vi "Initialize.vi"(8 "error in (no error)":errorcluster caption="错误输入（无错误）", 11 "Generic输入":refnum<class "Generic.lvclass">) -> (0 "error out":errorcluster caption="错误输出", 3 "Generic输出":refnum<class "Generic.lvclass">)   [LabVIEW 2013, in "Hierarchy Framework.lvlib" / "Generic.lvclass"]
uses:
  Generic.lvclass
  Generic.lvclass/Generic.ctl
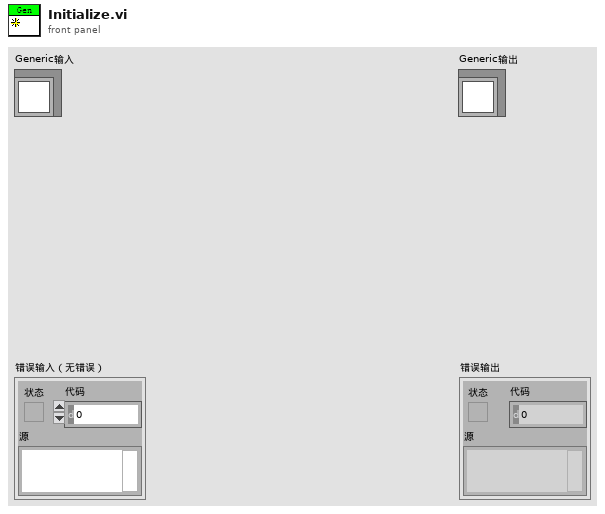
[diagram p1: front panel]
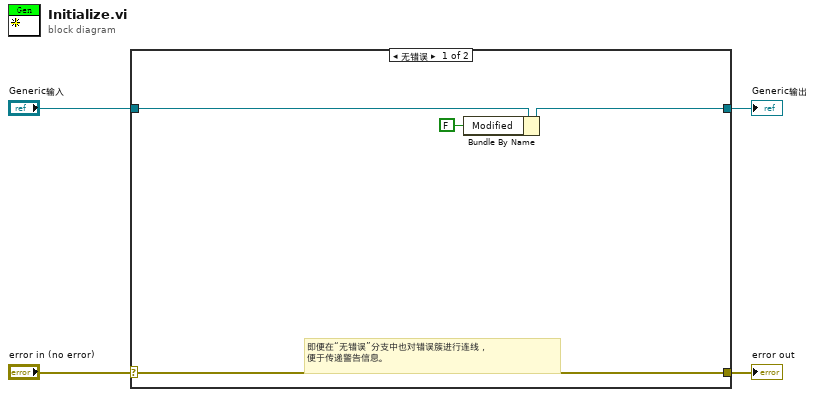
[diagram p0: block diagram]
diagram:
  n1 = case shown="无错误" "error in (no error)" {
    selector: "error in (no error)" -> [w7 w10]
    tunnel: [w7 w10] -> w3
    tunnel: [w6 w9] -> w1
    tunnel: "Generic输入" -> [w8 w9]
    frame No Error {
      # "即便在“无错误”分支中也对错误簇进行连线，\n便于传递警告信息。"
      n2 = Bundle By Name(cluster=w8, "Modified"=FALSE) -> (w6:refnum<class "Generic.lvclass">)
    }
    frame Error {
    }
  }
  "error out" <- w3
  "Generic输出" <- w1
